vi "PositionDifference.vi"(1 "(x,y)":T1, 2 "(x1,y1)":T1) -> (5 "(x-x1,y-y1)":T1)   [LabVIEW 2017]
uses:
  <vilib>/Utility/miscctls.llb/LVPositionTypeDef.ctl
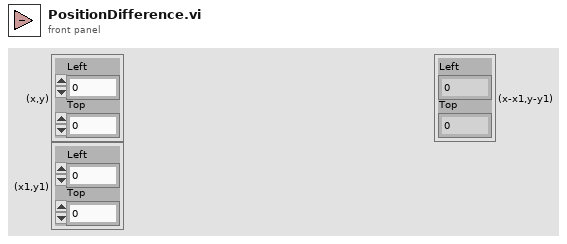
[diagram p1: front panel]
types:
  T1 = typedef "LVPositionTypeDef.ctl" = cluster{"Left":i32, "Top":i32}
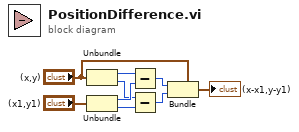
[diagram p0: block diagram]
diagram:
  n1 = Unbundle("(x,y)") -> ("Left"=w8:i32, "Top"=w6:i32)
  n2 = Unbundle("(x1,y1)") -> ("Left"=w7:i32, "Top"=w5:i32)
  n3 = Subtract(x=w8, y=w7) -> (x-y=w3:i32)
  n4 = Subtract(x=w6, y=w5) -> (x-y=w2:i32)
  n5 = Bundle(cluster="(x,y)", "Left"=w3, "Top"=w2) -> (→"(x-x1,y-y1)":T1)
